vi "Method.vi"(4 "Input B":refnum<class "Abs_Numeric.lvclass">, 5 "Input A":T1) -> (1 "Result":T1)   [LabVIEW 2021, in "Subtract_U16.lvclass"]
uses:
  Subtract_U16.lvclass
  Abs Type.ctl
  Abs_Types/U16 Integer/Abs_U16 Integer.lvclass
  Abs_Types/Numeric/Abs_Numeric.lvclass
  C:/Users/Tim/Documents/LabVIEW/2021/Data Classes/Source/Functions/Support/Two Terminal/U16/AbsFunc_Two Term_U16.lvclass
  C:/Users/Tim/Documents/LabVIEW/2021/Data Classes/Source/Abs_Types/U16 Integer/Abs_U16 Integer.lvclass
  Support/Two Terminal/U16/AbsFunc_Two Term_U16.lvclass/AbsFunc_Two Term_U16.ctl
  Support/Two Terminal/U16/Properties/Write Numeric A.vi
  Support/Two Terminal/U16/Properties/Write Numeric B.vi
  Subtract_U16.lvclass/Subtract_U16.ctl
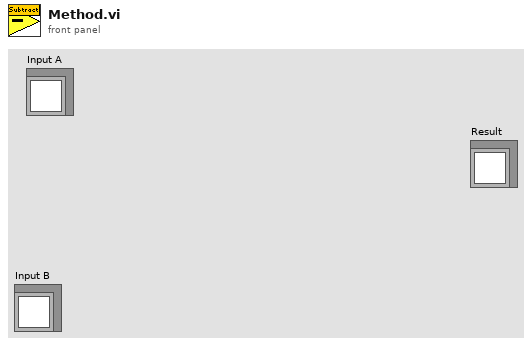
[diagram p1: front panel]
types:
  T1 = typedef "Subtract_U16.lvclass/Abs Type.ctl" = refnum<class "Abs_U16 Integer.lvclass">
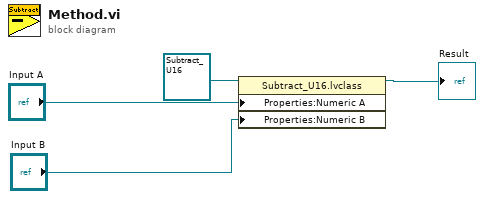
[diagram p0: block diagram]
diagram:
  n1 = property class="Subtract_U16.lvclass"(reference=refnum<class "Subtract_U16.lvclass"> refnum ("Subtract_DBL.lvclass"), "Properties:Numeric A"="Input A", "Properties:Numeric B"="Input B") -> (reference out=→"Result":refnum<class "Subtract_U16.lvclass">)  [unwired: 1 in, 1 out]
